vi "GAS_DETECTOR.vi"() -> (0 "Waveform Chart":dbl(graph), 1 "Gas Leakage Level Indicator":dbl)   [LabVIEW 2014]
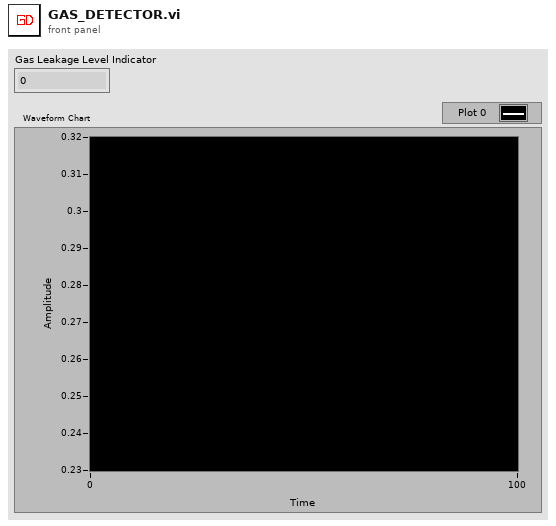
[diagram p1: front panel]
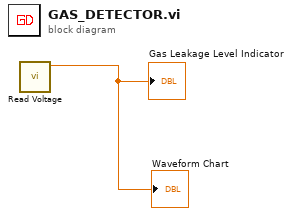
[diagram p0: block diagram]
diagram:
  n1 = call "Read Voltage.vi"() -> ("voltage"=→"Gas Leakage Level Indicator" →"Waveform Chart":dbl)  [unwired: 6 in, 1 out]
